vi "GetLayoutInfo.vi"(8 "error in (no error)":errorcluster, 11 "Column in":refnum<class "Column.lvclass">) -> (0 "error out":errorcluster, 2 "Layout cluster":T1, 3 "Column out":refnum<class "Column.lvclass">)   [LabVIEW 2013, in "Column.lvclass"]
doc: "Used by Layout dialog. Column name, background color, width, and isDisplayed? array are read for display in the Layout editing dialog. This is not the full set of appearances; GetAppearance.vi should be used to read name, width, and background and text colors."
uses:
  Column.lvclass
  TypeDefs/ColumnLayoutCluster.ctl
  Column.lvclass/Column.ctl
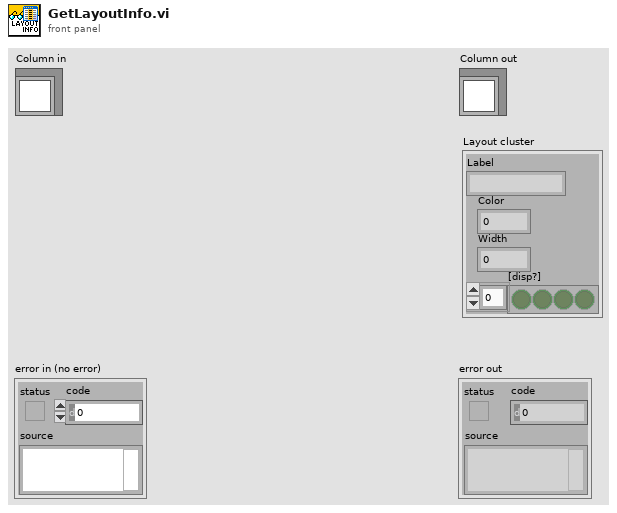
[diagram p1: front panel]
types:
  T1 = typedef "ColumnLayoutCluster.ctl" = cluster{"Label":string, "Color":u32, "Width":u32, "[disp?]":bool[]}
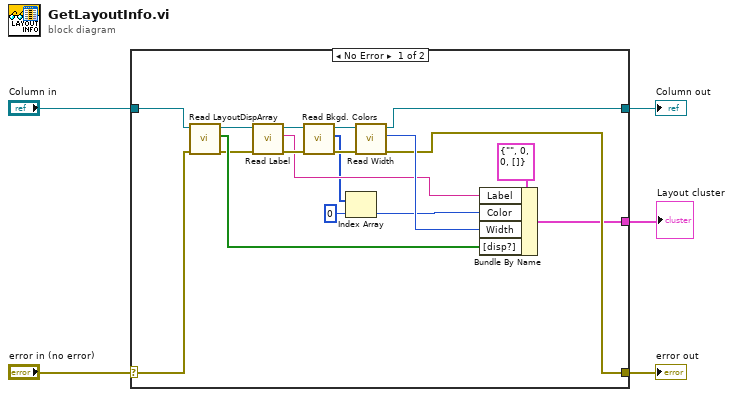
[diagram p0: block diagram]
diagram:
  n1 = case shown="No Error" "error in (no error)" {
    selector: "error in (no error)" -> [w23 w25]
    tunnel: [w8 w25] -> w4
    tunnel: [w14 w24] -> w2
    tunnel: "Column in" -> [w22 w24]
    tunnel: [w7 _] -> w1
    frame No Error {
      n2 = call "Read LayoutDispArray.vi"("error in (no error)"=w23, "Column in"=w22) -> ("error out"=w19:errorcluster, "Layout disp? array"=w21:bool[], "Column out"=w15:refnum<class "Column.lvclass">)  [unwired: 7 in]
      n3 = call "Read Label.vi"("error in (no error)"=w19, "Column in"=w15) -> ("error out"=w18:errorcluster, "Label"=w12:string, "Column out"=w20:refnum<class "Column.lvclass">)  [unwired: 7 in]
      n4 = call "Read Bkgd. Colors.vi"("error in (no error)"=w18, "Column in"=w20) -> ("error out"=w16:errorcluster, "Bkgd. Colors"=w11:u32[], "Column out"=w17:refnum<class "Column.lvclass">)  [unwired: 7 in]
      n5 = Index Array(array=w11, index=0) -> (element=w10:u32)
      n6 = call "Read Width.vi"("error in (no error)"=w16, "Column in"=w17) -> ("error out"=w8:errorcluster, "Width"=w13:u32, "Column out"=w14:refnum<class "Column.lvclass">)  [unwired: 7 in]
      n7 = Bundle By Name(cluster=T1 {"Label"="", "Color"=0, "Width"=0, "[disp?]"=[]} ("Layout cluster 2"), "Label"=w12, "Color"=w10, "Width"=w13, "[disp?]"=w21) -> (w7:T1)
    }
    frame Error {
    }
  }
  "error out" <- w4
  "Column out" <- w2
  "Layout cluster" <- w1
